vi "Write False.vi"   [LabVIEW 2019, in "LabPack.lvlib" / "Writer.lvclass"]
doc: "Writes and encodes a False boolean to the MessagePack binary data format."
uses:
  Writer.lvclass
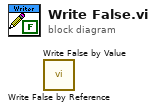
[diagram p0: block diagram]
diagram:
  n1 = call "Write False by Reference.vi"() -> ()  [unwired: 10 in, 2 out]
  n2 = call "Write False by Value.vi"() -> ()  [unwired: 10 in, 2 out]
